vi "Check Sum.vi"(8 "error in (no error)":errorcluster, 11 "string in":string) -> (0 "error out":errorcluster, 2 "string out":string, 3 "No Parse":bool)   [LabVIEW 2011]
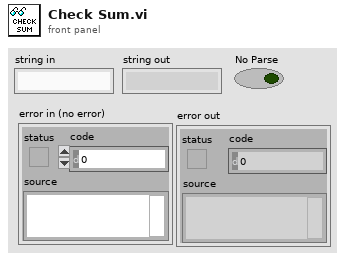
[diagram p1: front panel]
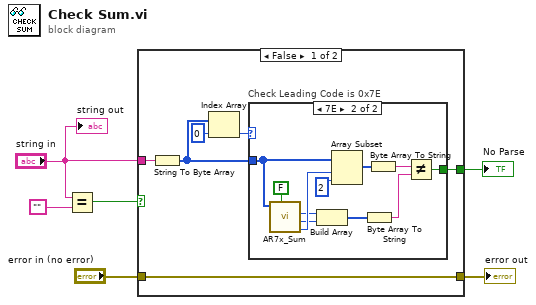
[diagram p0: block diagram]
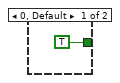
[diagram p2: hidden frame]
diagram:
  n1 = Equal?(x="string in", y="") -> (x = y?=w3:bool)
  n2 = case shown="False" w3 {
    selector: w3 -> [_ w26]
    tunnel: [w11 w26] -> w6
    tunnel: "string in" -> [w12 _]
    tunnel: "error in (no error)" -> [w7 w25]
    tunnel: [w7 w25] -> w1
    frame False {
      n3 = String To Byte Array(string=w12) -> (unsigned byte array=w9:u8[])
      n4 = Index Array(array=w9, index=0) -> (element=w8:u8)
      n5 = case "Check Leading Code is 0x7E" shown="7E" w8 {
        tunnel: w9 -> [_ w15]
        tunnel: [TRUE w14] -> w11
        frame 0, Default {
        }
        frame 126 {
          n6 = call "AR7x_Sum.vi"("output"=FALSE, "Cmd In"=w15) -> ("Length"=w20:u8, "SUM"=w18:u8, "XOR"=w17:u8)  [unwired: 6 in, 1 out]
          n7 = Build Array(w17, w18) -> (w22:u8[])
          n8 = Array Subset(array=w15, index=w20, length=2) -> (w21:u8[])
          n9 = Byte Array To String(unsigned byte array=w22) -> (string=w24:string)
          n10 = Byte Array To String(unsigned byte array=w21) -> (string=w23:string)
          n11 = Not Equal?(x=w23, y=w24) -> (x != y?=w14:bool)
        }
      }
    }
    frame True {
    }
  }
  "No Parse" <- w6
  "error out" <- w1
  "string out" <- "string in"
